vi "Gaincont.vi"(11 "Array":cdb[](array[numeric])) -> (3 "out":cdb[](array[numeric]))   [LabVIEW 2013]
uses:
  <vilib>/imath/engines/lvmath2/RunTimeEngine/ErrorHandling/NIMS_Finalize Error.vi
  <vilib>/imath/engines/lvmath2/RunTimeEngine/Managers/WorkSpace/UID Generator.vi
  <vilib>/imath/engines/lvmath2/RunTimeEngine/Managers/SymbolTable/Clear UID.vi
  <vilib>/imath/engines/lvmath2/RunTimeEngine/NodeEndStatement/NIMS_NodeEndStatement_Output.vi
  <instcachedir>/0/NIMS_NodeEndStatement_Output_53EC0D466D134D7ABD903AC30B43404B.lvgen/NIMS_NodeEndStatement_Output_53EC0D466D134D7ABD903AC30B43404B_000.vi
  LabVIEW Data/MathScriptVIs/MCStatic_31879994332_a259f4b8c64d073e3eb5702aefffdb1b.vi
  <instcachedir>/0/MCStatic_31879994332_a259f4b8c64d073e3eb5702aefffdb1b_668ED92A25C4486A88D3FE903AA8F216.lvgen/MCStatic_31879994332_a259f4b8c64d073e3eb5702aefffdb1b_668ED92A25C4486A88D3FE903AA8F216_000.vi
  <vilib>/imath/engines/lvmath2/RunTimeEngine/RunTimeType/NIMS_RunTimeType_From StrictType (excl LVString).vi
  <instcachedir>/0/NIMS_RunTimeType_From StrictType (excl LVString)_4DEE718D6EB74582AA20236969C084FC.lvgen/NIMS_RunTimeType_From StrictType (excl LVString)_4DEE718D6EB74582AA20236969C084FC_000.vi
  <vilib>/imath/engines/lvmath2/RunTimeEngine/LocalVariableDefStatement/MC_LocalVariableDefStatement_Display.vi
  MATLAB_func/gain_synch.m
  <vilib>/imath/engines/lvmath2/RunTimeEngine/Managers/SymbolTable/NIMS_WorkSpace.lvlib
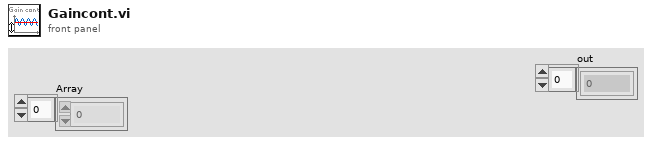
[diagram p1: front panel]
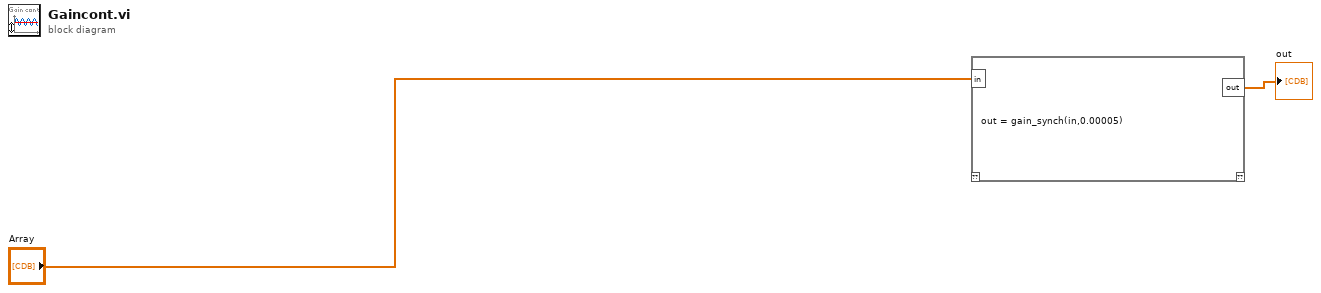
[diagram p0: block diagram]
diagram:
  n1 = mathscript code="out = gain_synch(in,0.00005)"("in"="Array") -> ("out"=→"out":cdb[])  [unwired: 1 in, 1 out]
